vi "CRYMouse.vi"() -> (1 "WinName":string, 4 "KeyState":bool[](array[boolean]), 5 "XPos":i32, 6 "YPos":i32, 7 "Button State latch":bool[](array[boolean]), 8 "Current Button State":bool[](array[boolean]))   [LabVIEW 2013]
uses:
  user.lib/Lvtoolbox DLL.dll
panel:
  # "Mouse Magic"
  # "left button"
  # "Mid button"
  # "right button"
  # "left button"
  # "Mid button"
  # "right button"
  # "left shift"
  # "right shift"
  # "left control"
  # "right control"
  # "LabVIEW Toolbox v1.3\nDanny Lauwers\n(c) 1994-1996"
  # "left menu (win95 keyboard)"
  # "right menu (win95 keyboard)"
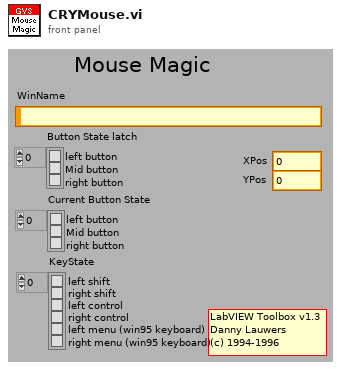
[diagram p1: front panel]
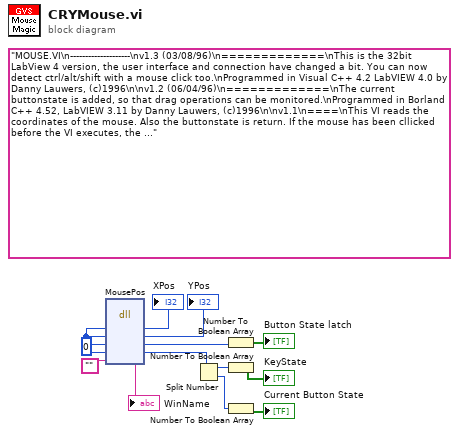
[diagram p0: block diagram]
diagram:
  w12 = 0
  (unwired) "MOUSE.VI\n--------------------\nv1.3 (03/08/96)\n=============\nThis is the 32bit LabView 4 version, the user interface and connection have changed a bit. You can now detect ctrl/alt/shift with a mouse click too.\nProgrammed in Visual C++ 4.2 LabVIEW 4.0 by Danny Lauwers, (c)1996\n\nv1.2 (06/04/96)\n=============\nThe current buttonstate is added, so that drag operations can be monitored.\nProgrammed in Borland C++ 4.52, LabVIEW 3.11 by Danny Lauwers, (c)1996\n\nv1.1\n====\nThis VI reads the coordinates of the mouse. Also the buttonstate is return. If the mouse has been cllicked before the VI executes, the mousebutton operation is still detected. The foor Boolean on the screen indicate the current position of the mouse and the button state. The name of the window is also return, and can be used by windowMagic to hide, move or set focus to the window.\nProgrammed in Borland C++ 4.0, LabVIEW 3.1  by Danny Lauwers,  (c)1994\n\n\nYou can use this VI in you program as long as you keep this text with it and do not cleam that you wrote it. Have fun with it !!\n\nI am not responsible for any crashes from this program, but for now it seems very stable.\n\nDanny Lauwers\ndlauwers@innet.be"
  n1 = dll-call lib="D:/LabView_Project/CRY6181/user.lib/lvtoolbox DLL.dll" fn="MousePos"("Xpos"=w12, "Ypos"=w12, "BS"=w12, "CBS"=w12, "WinName"="") -> ("Xpos"=→"XPos":i32, "Ypos"=→"YPos":i32, "BS"=w3:i32, "CBS"=w2:i32, "WinName"=→"WinName":string)  [unwired: 3 in, 3 out]
  n2 = Split Number(x=w2) -> (hi(x)=w7:u16, lo(x)=w1:u16)
  n3 = Number To Boolean Array(number=w3) -> (Boolean array=→"Button State latch":bool[])
  n4 = Number To Boolean Array(number=w7) -> (Boolean array=→"KeyState":bool[])
  n5 = Number To Boolean Array(number=w1) -> (Boolean array=→"Current Button State":bool[])
